vi "Read IL Action.vi"(11 "Interlock Chain in":refnum<class "Interlock Chain.lvclass">) -> (2 "IL Action Override":refnum<class "IL Action.lvclass">[](array[class]), 3 "Interlock Chain out":refnum<class "Interlock Chain.lvclass">)   [LabVIEW 2015, in "Interlocks.lvlib" / "Interlock Chain.lvclass"]
uses:
  Interlock Chain.lvclass
  IL Action/IL Action.lvclass
  Interlock Chain.lvclass/Interlock Chain.ctl
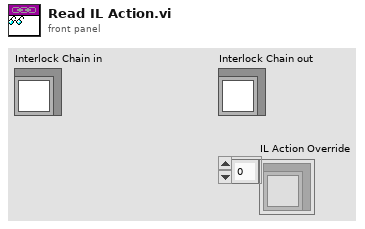
[diagram p1: front panel]
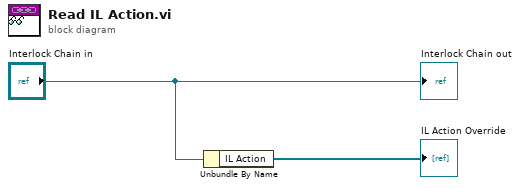
[diagram p0: block diagram]
diagram:
  n1 = Unbundle By Name("Interlock Chain in") -> ("IL Action"=→"IL Action Override":refnum<class "IL Action.lvclass">[])
  "Interlock Chain out" <- "Interlock Chain in"
